vi "csm_lumikki_instron_moveToSetpoint_poller.vi"() -> ()   [LabVIEW 2009]
panel:
  out "setpoint":dbl
  out "channel":i32
  out "newSetpointCommandArrived":bool
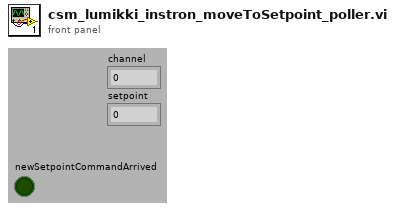
[diagram p1: front panel]
types:
  T1 = cluster{"Name":string, "Type":i32, "SI Full Scale":dbl, "Full Scale":dbl, "Units String":string, "Display Format":string, "Gauge Length":dbl}[][]
  T2 = cluster{"Device ID":i32, "Device Name":string, "Device Type":i32}[]
  T3 = cluster{"Double":dbl, "Double":dbl, "setpointTime":dbl, "setpointTime":dbl}
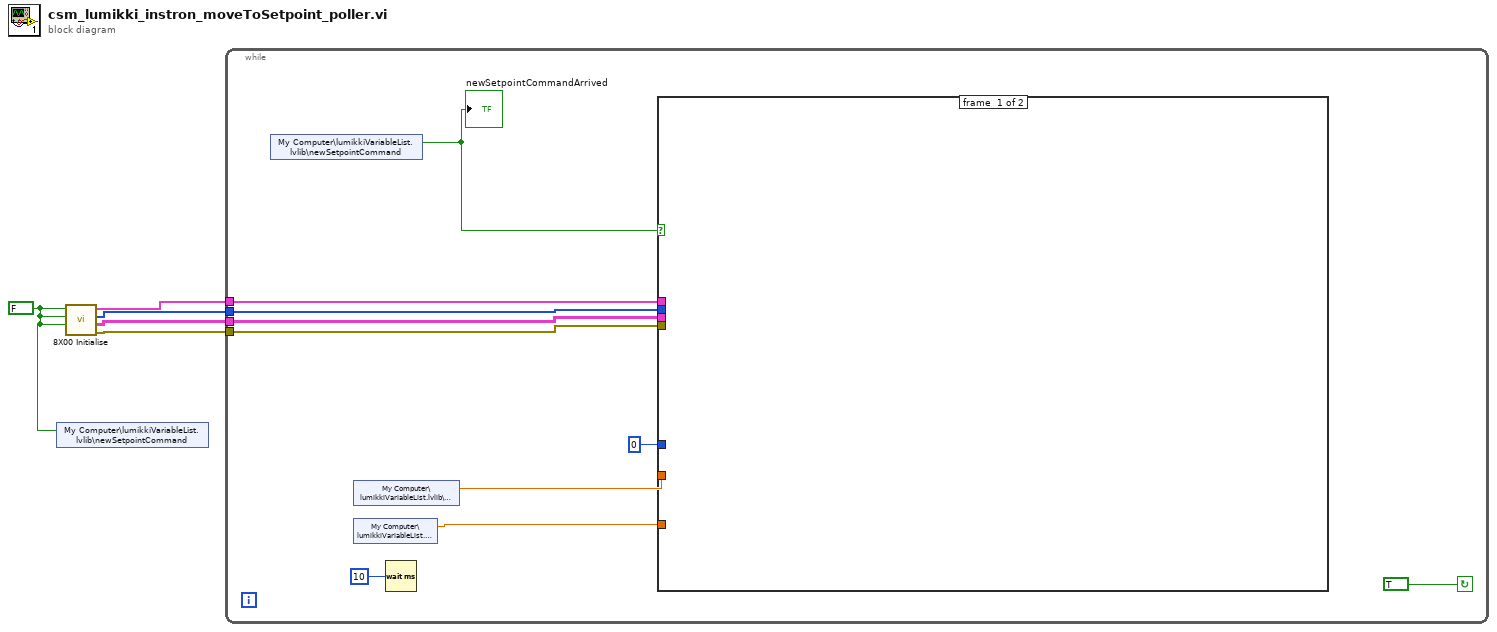
[diagram p0: block diagram]
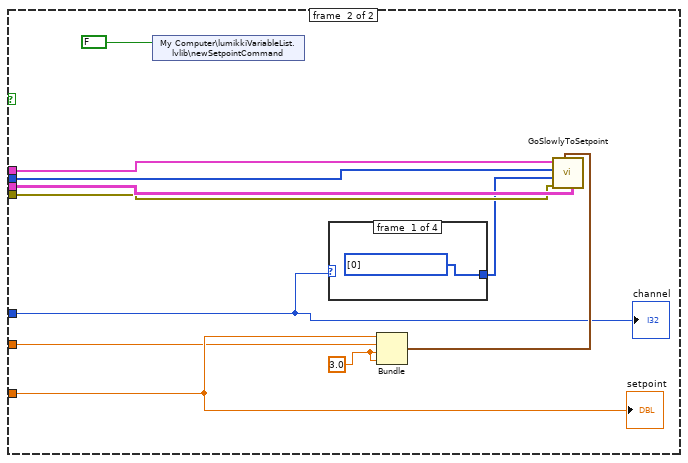
[diagram p2: hidden frame]
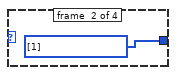
[diagram p3: hidden frame]
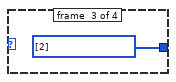
[diagram p4: hidden frame]
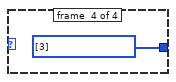
[diagram p5: hidden frame]
diagram:
  w1 = FALSE ("Create Console? (T)")
  n1 = shared-variable "My Computer\\lumikkiVariableList.lvlib\\newSetpointCommand"(w1) -> ()  [unwired: 1 in, 1 out]
  n2 = call "8X00 Initialise.vi"("Reset?"=w1, "Create DVM? (T)"=w1, "Create Console? (T)"=w1) -> ("error out"=w2:errorcluster, "Channel Data"=w3:T1, "Axis Selector"=w4:i32[], "Axis Information"=w5:T2)  [unwired: 1 in]
  n3 = while {
    tunnel: w5 -> [w13]
    tunnel: w4 -> [w12]
    tunnel: w3 -> [w11]
    tunnel: w2 -> [w10]
    stop <- TRUE continue-if-true
    n4 = shared-variable "My Computer\\lumikkiVariableList.lvlib\\newSetpointCommand"() -> (w8:bool)  [unwired: 1 in, 1 out]
    "newSetpointCommandArrived" <- w8
    n5 = shared-variable "My Computer\\lumikkiVariableList.lvlib\\setpointTime"() -> (w6:dbl)  [unwired: 1 in, 1 out]
    n6 = shared-variable "My Computer\\lumikkiVariableList.lvlib\\setpoint"() -> (w9:dbl)  [unwired: 1 in, 1 out]
    n7 = Wait (ms)(milliseconds to wait=u32 10) -> ()  [unwired: 1 out]
    n8 = case shown="True" w8 {
      tunnel: w13 -> [_ w25]
      tunnel: w12 -> [_ w24]
      tunnel: w11 -> [_ w23]
      tunnel: w10 -> [_ w22]
      tunnel: w9 -> [_ w26]
      tunnel: 0 ("channelInt") -> [_ w19]
      tunnel: w6 -> [_ w17]
      frame #0 {
      }
      frame #1 {
        w16 = 3.0 ("setpointTime")
        n9 = shared-variable "My Computer\\lumikkiVariableList.lvlib\\newSetpointCommand"(FALSE ("newSetpointCommand")) -> ()  [unwired: 1 in, 1 out]
        n10 = case shown="4" w19 {
          tunnel: [w27 w28 w29 w30] -> w21
          frame #0 {
            w27 = u16[] [0] items=["Channel 1", "Channel 2", "Channel 3", "Channel 4"] ("Choose channel to apply\nthe setpoint")
          }
          frame #1 {
            w28 = u16[] [1] items=["Channel 1", "Channel 2", "Channel 3", "Channel 4"] ("Choose channel to apply\nthe setpoint")
          }
          frame #2 {
            w29 = u16[] [2] items=["Channel 1", "Channel 2", "Channel 3", "Channel 4"] ("Choose channel to apply\nthe setpoint")
          }
          frame #3 {
            w30 = u16[] [3] items=["Channel 1", "Channel 2", "Channel 3", "Channel 4"] ("Choose channel to apply\nthe setpoint")
          }
        }
        n11 = Bundle("Double"=w26, "Double"=w17, "setpointTime"=w16, "setpointTime"=w16) -> (w20:T3)  [unwired: 1 in]
        n12 = call "GoSlowlyToSetpoint.vi"("Channel Data"=w23, "Input cluster"=w20, "error in (no error)"=w22, "Channels"=w21, "Axis Selector"=w24, "Axis Information"=w25) -> ()  [unwired: 2 in, 4 out]
        "channel" <- w19
        "setpoint" <- w26
      }
    }
  }
